vi "S2C_FORNAX_Proc_FormatViper.vi"(8 "Error In":errorcluster, 10 "Parameter":string, 11 "Command":string) -> (0 "Error Out":errorcluster, 3 "VipMsg":string[](array[string]))   [LabVIEW 2015]
uses:
  S2C_FORNAX_Proc_Globals.vi
  <vilib>/Utility/file.llb/Read Delimited Spreadsheet (string).vi
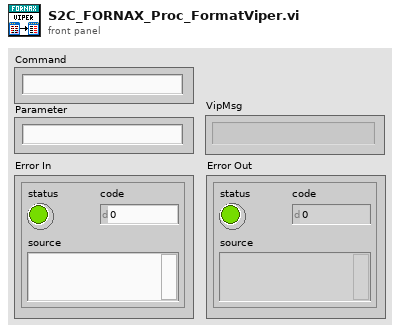
[diagram p1: front panel]
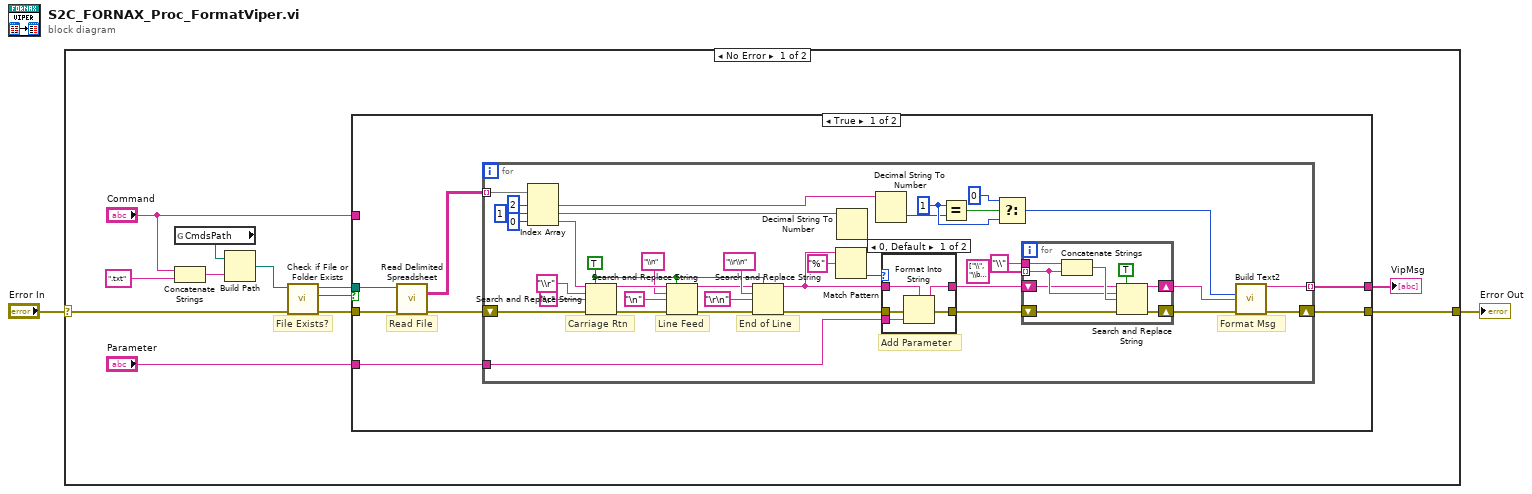
[diagram p0: block diagram]
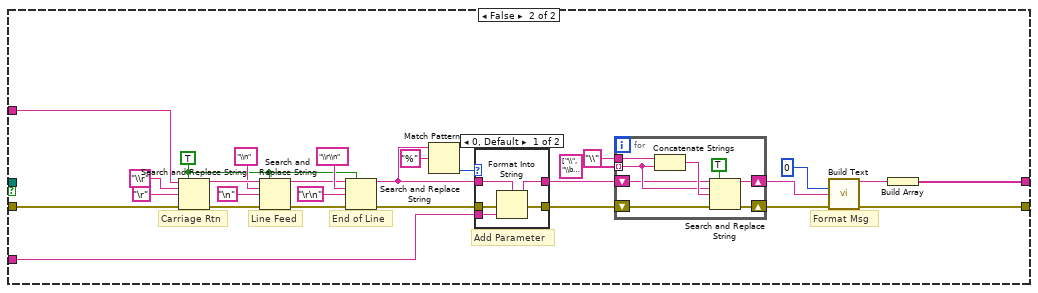
[diagram p3: hidden frame]
diagram:
  n1 = case shown="No Error" "Error In" {
    selector: "Error In" -> [w10 w117]
    tunnel: [w11 w117] -> w1
    frame No Error {
      # "File Exists?"
      n2 = global read "S2C_FORNAX_Proc_Globals.vi" "CmdsPath"() -> (w12:path)
      n3 = Concatenate Strings("Command", ".txt" ("string")) -> (w13:string)
      n4 = Build Path(base path=w12, name or relative path=w13) -> (appended path=w9:path)
      n5 = call <vilib>:"Check if File or Folder Exists.vi"("error in (no error)"=w10, "path"=w9) -> ("error out"=w8:errorcluster, "file or folder exists?"=w7:bool, "dup path"=w6:path)  [unwired: 7 in]
      n6 = case shown="True" w7 {
        tunnel: [w19 w101] -> w11
        tunnel: w8 -> [w17 w75]
        tunnel: w6 -> [w18 _]
        tunnel: "Parameter" -> [w16 w100]
        tunnel: [w15 w76] -> w4
        tunnel: "Command" -> [_ w74]
        frame True {
          # "Read File"
          n7 = call-poly <vilib>:"Read Delimited Spreadsheet.vi"("file path (dialog if empty)"=w18, "error in (no error)"=w17) -> ("all rows"=w21:string[][], "error out"=w20:errorcluster)  [unwired: 8 in, 4 out]
          n8 = for {
            tunnel: w21 -> [w58] mode=indexing
            shift-right: [w23] -> w19
            shift-left: w20 -> [w49]
            tunnel: w16 -> [w30]
            tunnel: [w22] -> w15 mode=indexing
            w39 = i8 1 ("x")
            w42 = TRUE ("replace all? (F)")
            # "Add Parameter"
            # "Format Msg"
            # "End of Line"
            # "Line Feed"
            # "Carriage Rtn"
            n9 = Index Array(array=w58, index #1=2 ("index"), index #2=1 ("index"), index #3=0 ("index")) -> (element #1=w41:string, element #2=w40:string, element #3=w47:string)
            n10 = Search and Replace String(replace all?=w42, input string=w47, search string="\\r", replace string="\r", error in=w49) -> (result string=w53:string, error out=w50:errorcluster)  [unwired: 5 out]
            n11 = Search and Replace String(replace all?=w42, input string=w53, search string="\\n", replace string="\n", error in=w50) -> (result string=w43:string, error out=w44:errorcluster)  [unwired: 5 out]
            n12 = Search and Replace String(replace all?=w42, input string=w43, search string="\\r\\n", replace string="\r\n", error in=w44) -> (result string=w31:string, error out=w32:errorcluster)  [unwired: 5 out]
            n13 = Match Pattern(string=w31, regular expression="%") -> (offset past match=w29:i32)  [unwired: 4 out]
            n14 = Decimal String To Number(string=w40) -> ()  [unwired: 4 out]
            n15 = Decimal String To Number(string=w41) -> (number=w36:i32)  [unwired: 3 out]
            n16 = case shown="0, Default" w29 {
              tunnel: w32 -> [w63 w64]
              tunnel: w31 -> [w62 w65]
              tunnel: w30 -> [w61 _]
              tunnel: [w60 w65] -> w28
              tunnel: [w59 w64] -> w27
              frame 0, Default {
                n17 = Format Into String(format string=w62, error in=w63, w61) -> (resulting string=w60:string, error out=w59:errorcluster)  [unwired: 1 in]
              }
              frame -1 {
              }
            }
            n18 = Equal?(x=w39, y=w36) -> (x = y?=w37:bool)
            n19 = Select(t=i8 0 ("x"), s=w37, f=w39) -> (s? t:f=w25:i8)
            n20 = for {
              tunnel: string[] ["\\", "\\b", "\\f", "\\n", "\\r", "\\t", "\\v", "'", "\""] -> [w72] mode=indexing
              shift-right: [w71] -> w24
              shift-left: w28 -> [w70]
              shift-right: [w67] -> w26
              shift-left: w27 -> [w68]
              tunnel: "\\" ("string") -> [w66]
              n21 = Concatenate Strings(w66, w72) -> (w73:string)
              n22 = Search and Replace String(replace all?=TRUE ("replace all? (F)"), input string=w70, search string=w72, replace string=w73, error in=w68) -> (result string=w71:string, error out=w67:errorcluster)  [unwired: 3 in, 2 out]
            }
            n23 = call "Build Text2"("ID"=w25, "Msg"=w24, "error in (no error)"=w26) -> ("Result"=w22:string, "error out"=w23:errorcluster)  [unwired: 11 in]
          }
        }
        frame False {
          w88 = TRUE ("replace all? (F)")
          # "Add Parameter"
          # "Format Msg"
          # "End of Line"
          # "Line Feed"
          # "Carriage Rtn"
          n24 = Search and Replace String(replace all?=w88, input string=w74, search string="\\r", replace string="\r", error in=w75) -> (result string=w96:string, error out=w93:errorcluster)  [unwired: 5 out]
          n25 = Search and Replace String(replace all?=w88, input string=w96, search string="\\n", replace string="\n", error in=w93) -> (result string=w89:string, error out=w90:errorcluster)  [unwired: 5 out]
          n26 = Search and Replace String(replace all?=w88, input string=w89, search string="\\r\\n", replace string="\r\n", error in=w90) -> (result string=w83:string, error out=w84:errorcluster)  [unwired: 5 out]
          n27 = Match Pattern(string=w83, regular expression="%") -> (offset past match=w82:i32)  [unwired: 4 out]
          n28 = case shown="0, Default" w82 {
            tunnel: w84 -> [w106 w107]
            tunnel: w83 -> [w105 w108]
            tunnel: w100 -> [w104 _]
            tunnel: [w103 w108] -> w81
            tunnel: [w102 w107] -> w80
            frame 0, Default {
              n29 = Format Into String(format string=w105, error in=w106, w104) -> (resulting string=w103:string, error out=w102:errorcluster)  [unwired: 1 in]
            }
            frame -1 {
            }
          }
          n30 = for {
            tunnel: string[] ["\\", "\\b", "\\f", "\\n", "\\r", "\\t", "\\v", "'", "\""] -> [w115] mode=indexing
            shift-right: [w114] -> w78
            shift-left: w81 -> [w113]
            shift-right: [w110] -> w79
            shift-left: w80 -> [w111]
            tunnel: "\\" ("string") -> [w109]
            n31 = Concatenate Strings(w109, w115) -> (w116:string)
            n32 = Search and Replace String(replace all?=TRUE ("replace all? (F)"), input string=w113, search string=w115, replace string=w116, error in=w111) -> (result string=w114:string, error out=w110:errorcluster)  [unwired: 3 in, 2 out]
          }
          n33 = call "Build Text"("ID"=i8 0 ("x"), "Msg"=w78, "error in (no error)"=w79) -> ("Result"=w99:string, "error out"=w101:errorcluster)  [unwired: 11 in]
          n34 = Build Array(w99) -> (w76:string[])
        }
      }
      "VipMsg" <- w4
    }
    frame Error {
    }
  }
  "Error Out" <- w1
